vi "ble_cmd_end_procedure.vi"(8 "error in (no error)":errorcluster, 11 "COM Bluegiga in":refnum<visa-resource-name>) -> (0 "error out":errorcluster, 3 "COM Bluegiga out":refnum<visa-resource-name>)   [LabVIEW 2013]
uses:
  type_def/message_class.ctl
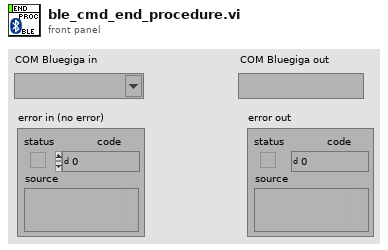
[diagram p1: front panel]
types:
  T1 = typedef "message_class.ctl" = u8
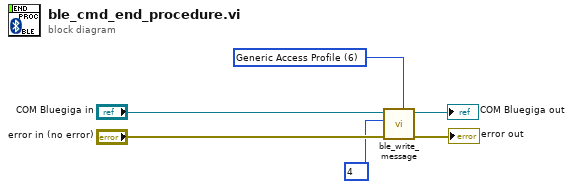
[diagram p0: block diagram]
diagram:
  w3 = T1 6 items=["System", "Persistent Store", "Attribute database", "Connection", "Attribute client", "Security Manager", "Generic Access Profile", "Hardware"] ("Command Class (System)")
  n1 = call "ble_write_message.vi"("Command Class (System)"=w3, "error in (no error)"="error in (no error)", "Message ID (0x00)"=u8 4, "COM Bluegiga in"="COM Bluegiga in") -> ("error out"=→"error out":errorcluster, "COM Bluegiga out"=→"COM Bluegiga out":refnum<visa-resource-name>)  [unwired: 5 in, 1 out]
